vi "ReadExperimentRunTotalChargeNode.vi"(8 "Error In":errorcluster, 11 "Experiment Run Node In":refnum<k20>) -> (0 "Error Out":errorcluster, 2 "Experiment Run Total Charge (C)":T1, 3 "Experiment Run Node Out":refnum<k20>)   [LabVIEW 2012]
uses:
  ExperimentRunTotalCharge.ctl
  <vilib>/xml/NI_XML.lvlib
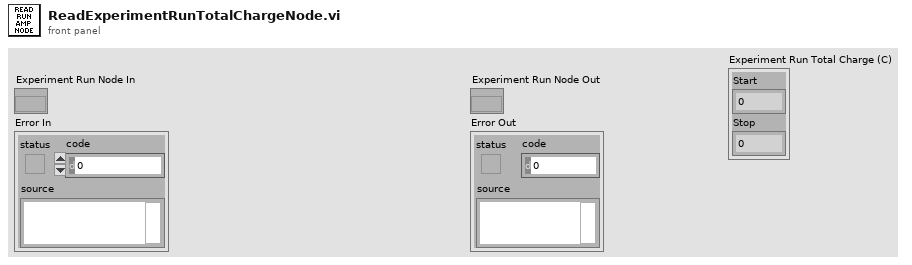
[diagram p1: front panel]
types:
  T1 = typedef "ExperimentRunTotalCharge.ctl" = cluster{"Start":dbl, "Stop":dbl}
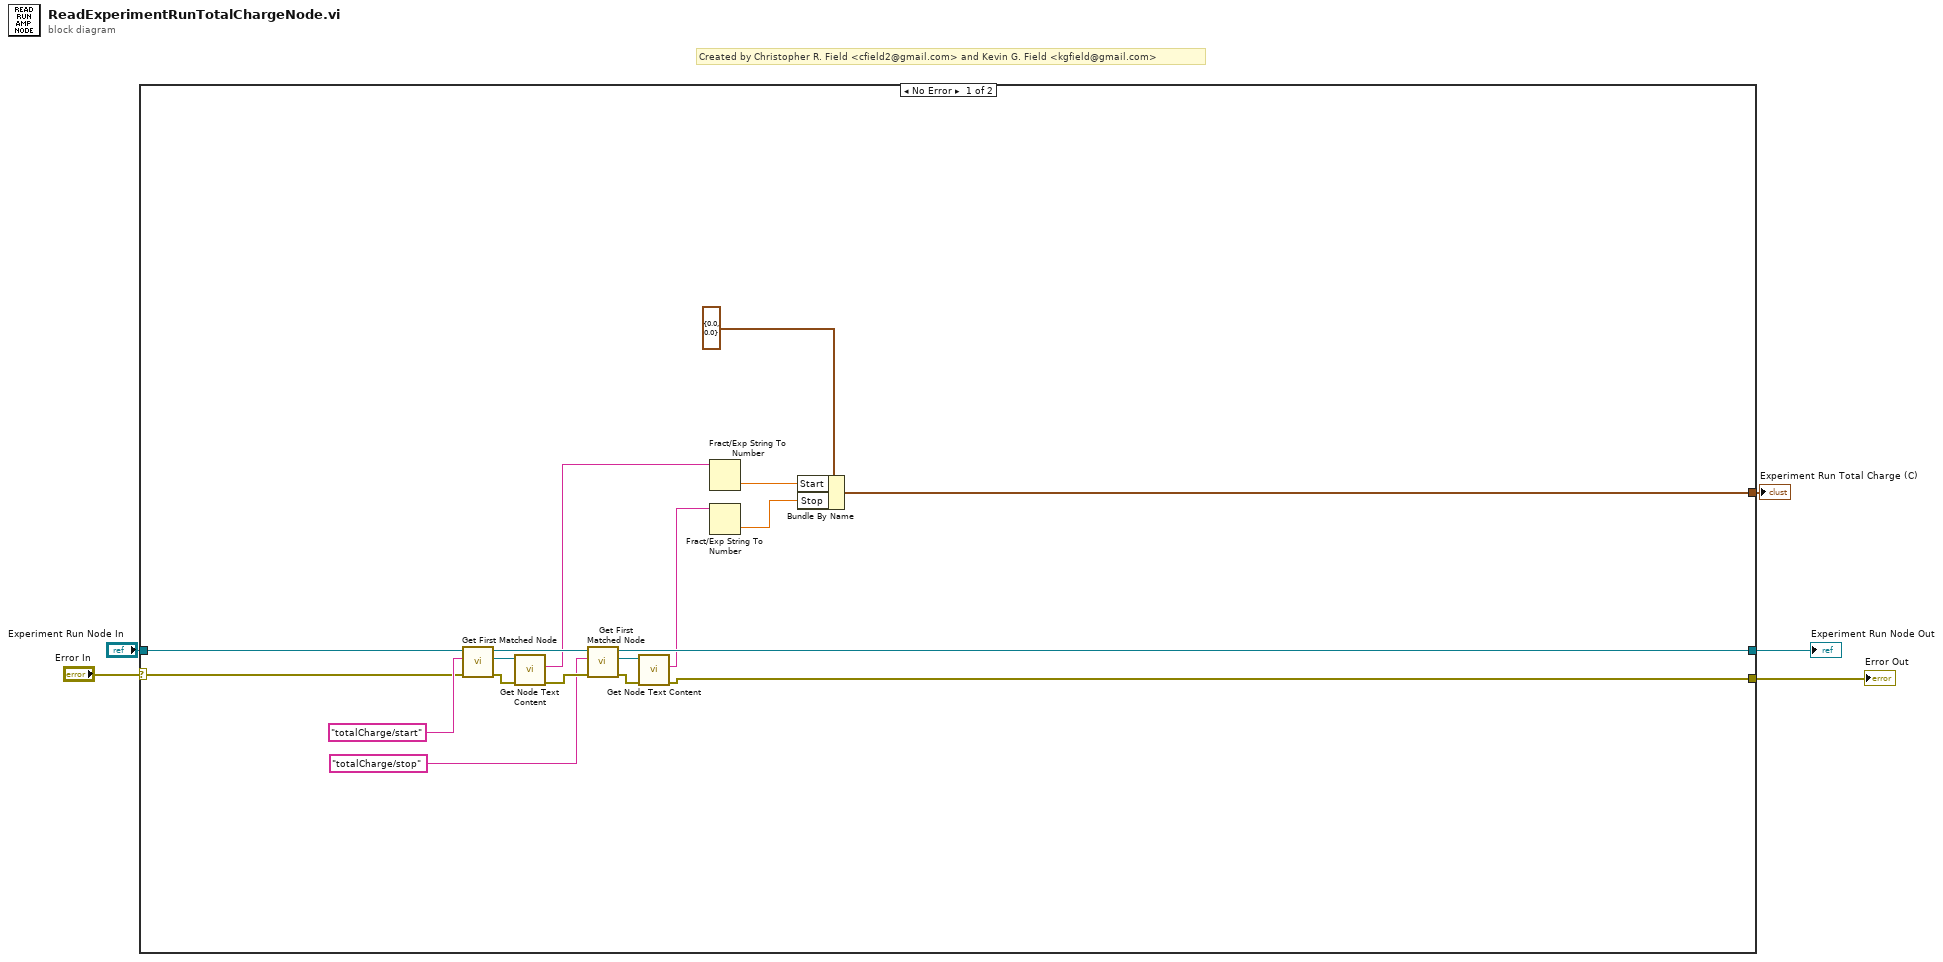
[diagram p0: block diagram]
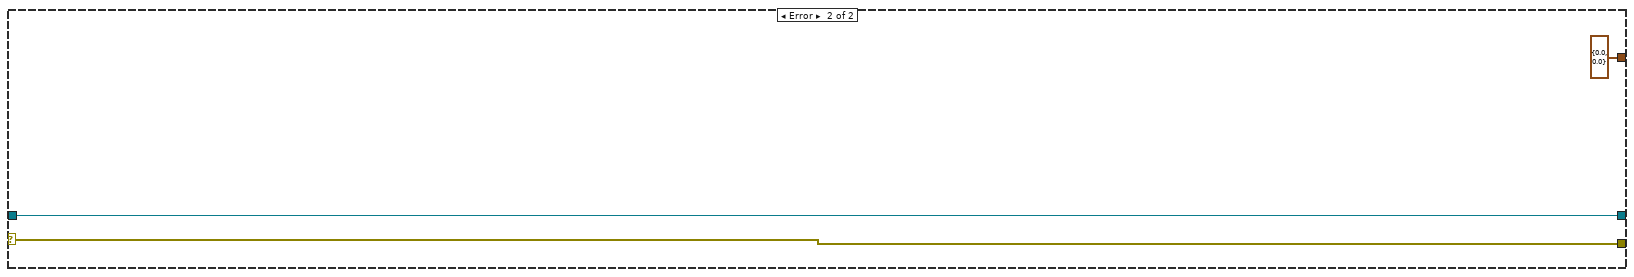
[diagram p2: hidden frame]
diagram:
  # "Created by Christopher R. Field <cfield2@gmail.com> and Kevin G. Field <kgfield@gmail.com>"
  n1 = case shown="No Error" "Error In" {
    selector: "Error In" -> [w12 w25]
    tunnel: "Experiment Run Node In" -> [w13 w26]
    tunnel: [w15 w26] -> w3
    tunnel: [w14 w25] -> w2
    tunnel: [w6 T1 {"Start"=0.0, "Stop"=0.0} ("Experiment Run Current (A)")] -> w1
    frame No Error {
      n2 = call <vilib>:"Get First Matched Node.vi"("error in (no error)"=w12, "XPath expression"="totalCharge/start", "node in"=w13) -> ("error out"=w21:errorcluster, "node result"=w22:refnum<k20>, "node out"=w20:refnum<k20>)  [unwired: 6 in]
      n3 = call <vilib>:"Get Node Text Content.vi"("error in (no error)"=w21, "node in"=w22) -> ("error out"=w19:errorcluster, "node text"=w11:string)  [unwired: 7 in, 1 out]
      n4 = call <vilib>:"Get First Matched Node.vi"("error in (no error)"=w19, "XPath expression"="totalCharge/stop", "node in"=w20) -> ("error out"=w16:errorcluster, "node result"=w17:refnum<k20>, "node out"=w15:refnum<k20>)  [unwired: 6 in]
      n5 = call <vilib>:"Get Node Text Content.vi"("error in (no error)"=w16, "node in"=w17) -> ("error out"=w14:errorcluster, "node text"=w10:string)  [unwired: 7 in, 1 out]
      n6 = Fract/Exp String To Number(string=w11) -> (number=w9:dbl)  [unwired: 3 in, 1 out]
      n7 = Fract/Exp String To Number(string=w10) -> (number=w8:dbl)  [unwired: 3 in, 1 out]
      n8 = Bundle By Name(cluster=T1 {"Start"=0.0, "Stop"=0.0} ("Experiment Run Current (A)"), "Start"=w9, "Stop"=w8) -> (w6:T1)
    }
    frame Error {
    }
  }
  "Experiment Run Node Out" <- w3
  "Error Out" <- w2
  "Experiment Run Total Charge (C)" <- w1
